vi "DEV Write User Data.vi"(7 "DataLen":i32, 9 "pWriteData":string, 10 "OffsetAddr":i32, 11 "DevHandle":i32) -> (1 "pWriteData out":string, 3 "function return":u8)   [LabVIEW 2010, in "usb_device.lvlib"]
doc: "unsigned char WINAPI DEV_WriteUserData(int DevHandle,int OffsetAddr,unsigned char *pWriteData,int DataLen);"
uses:
  usb_device.lvlib
  USB2XXX/trunk/USB2XXX/USB2XXX/vs2019/Release/USB2XXX.dll
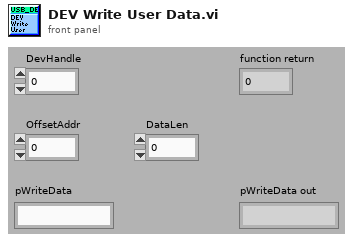
[diagram p1: front panel]
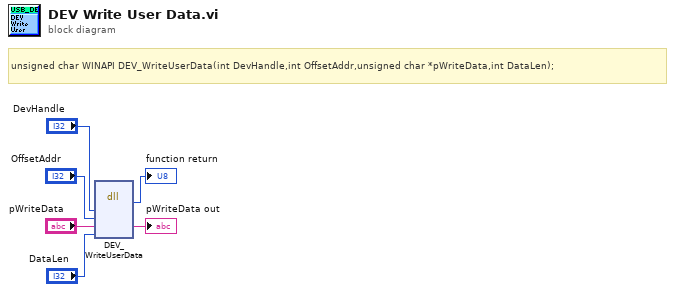
[diagram p0: block diagram]
diagram:
  # "unsigned char WINAPI DEV_WriteUserData(int DevHandle,int OffsetAddr,unsigned char *pWriteData,int DataLen);"
  n1 = dll-call lib="E:/Projects/USB2XXX/trunk/USB2XXX/USB2XXX/vs2019/Release/USB2XXX.*" fn="DEV_WriteUserData"("DevHandle"="DevHandle", "OffsetAddr"="OffsetAddr", "pWriteData"="pWriteData", "DataLen"="DataLen") -> (→"function return":u8, "pWriteData"=→"pWriteData out":string)  [unwired: 6 in, 2 out]
